vi "Bundle RT Configuration.vi"(8 "error in (no error)":errorcluster) -> (0 "error out":errorcluster, 3 "All Control Configuration Values":T1)   [LabVIEW 2018]
uses:
  controls/All Control Configuration Values.ctl
  controls/Control State.ctl
  controls/Raw Values.ctl
  controls/Control Configuration.ctl
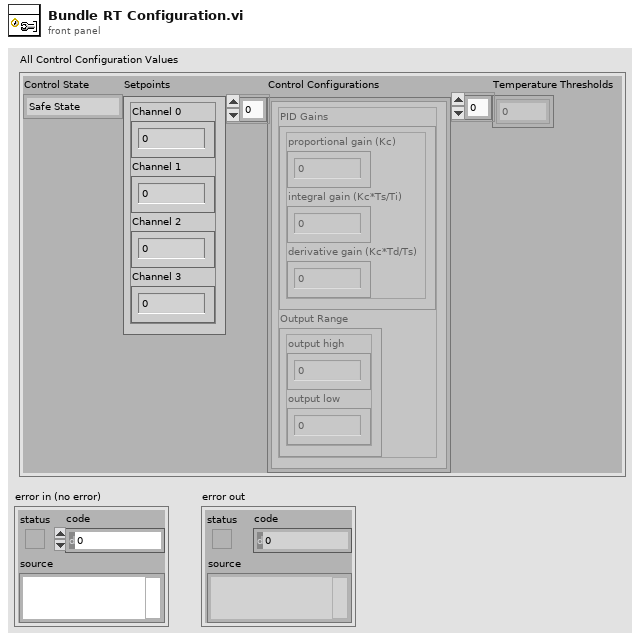
[diagram p1: front panel]
types:
  T1 = typedef "All Control Configuration Values.ctl" = cluster{"Control State":T2, "Setpoints":T3, "Control Configurations":T4[], "Temperature Thresholds":dbl[]}
  T2 = typedef "Control State.ctl" = enum16{"Safe State", "Control (PID)"}
  T3 = typedef "Raw Values.ctl" = cluster{"Channel 0":dbl, "Channel 1":dbl, "Channel 2":dbl, "Channel 3":dbl}
  T4 = typedef "Control Configuration.ctl" = cluster{"PID Gains":cluster{"proportional gain (Kc)":dbl, "integral gain (Kc*Ts/Ti)":dbl, "derivative gain (Kc*Td/Ts)":dbl}, "Output Range":cluster{"output high":dbl, "output low":dbl}}
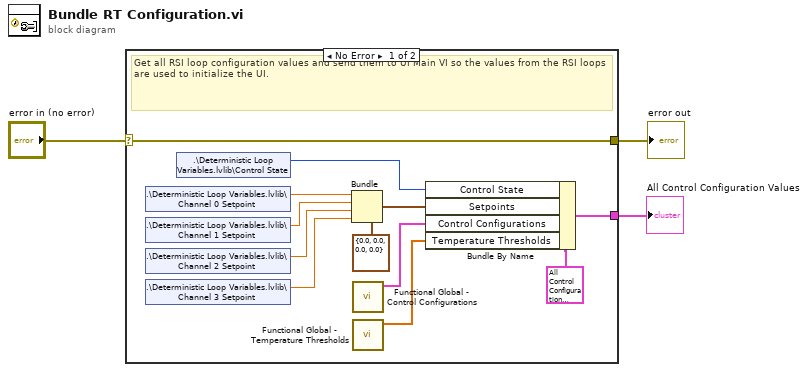
[diagram p0: block diagram]
diagram:
  n1 = case shown="No Error" "error in (no error)" {
    selector: "error in (no error)" -> [w13 w16]
    tunnel: [w13 w16] -> w2
    tunnel: [w14 _] -> w1
    frame No Error {
      # "Get all RSI loop configuration values and send them to UI Main VI so the values from the RSI loops are used to initialize the UI."
      n2 = shared-variable ".\\Deterministic Loop Variables.lvlib\\Channel 0 Setpoint"() -> (w7:dbl)  [unwired: 1 in, 1 out]
      n3 = shared-variable ".\\Deterministic Loop Variables.lvlib\\Channel 1 Setpoint"() -> (w6:dbl)  [unwired: 1 in, 1 out]
      n4 = shared-variable ".\\Deterministic Loop Variables.lvlib\\Channel 2 Setpoint"() -> (w5:dbl)  [unwired: 1 in, 1 out]
      n5 = shared-variable ".\\Deterministic Loop Variables.lvlib\\Channel 3 Setpoint"() -> (w4:dbl)  [unwired: 1 in, 1 out]
      n6 = shared-variable ".\\Deterministic Loop Variables.lvlib\\Control State"() -> (w8:T2)  [unwired: 1 in, 1 out]
      n7 = Bundle(cluster=T3 {"Channel 0"=0.0, "Channel 1"=0.0, "Channel 2"=0.0, "Channel 3"=0.0} ("Raw Values"), "Channel 0"=w7, "Channel 1"=w6, "Channel 2"=w5, "Channel 3"=w4) -> (w12:T3)
      n8 = call "Functional Global - Control Configurations.vi"() -> ("Control Configurations out"=w10:T4[])  [unwired: 11 in]
      n9 = call "Functional Global - Temperature Thresholds.vi"() -> ("Temperature Thresholds out"=w9:dbl[])  [unwired: 11 in]
      n10 = Bundle By Name(cluster=T1 {"Control State"=enum."Safe State", "Setpoints"={"Channel 0"=0.0, "Channel 1"=0.0, "Channel 2"=0.0, "Channel 3"=0.0}, "Control Configurations"=[], "Temperature Thresholds"=[]} ("All FPGA Configuration Values"), "Control State"=w8, "Setpoints"=w12, "Control Configurations"=w10, "Temperature Thresholds"=w9) -> (w14:T1)
    }
    frame Error {
      # "Error"
    }
  }
  "error out" <- w2
  "All Control Configuration Values" <- w1
